vi "pumpsec_new.vi"() -> ()   [LabVIEW 2015]
uses:
  BERTTA.dll
panel:
  out "mA":dbl format="%#_2g"
  out "params":dbl[](array[numeric])
  in  "Time":dbl[](array[numeric])=[4.0, 2.0, 0.0, 0.0, 0.0, 0.0, 0.0, 0.0, 0.0, 0.0]
  in  "Target":dbl[](array[numeric])=[10.0, 2.0, 0.0, 0.0, 0.0, 0.0, 0.0, 0.0, 0.0, 0.0]
  out "Scale":dbl
  in  "Port":i32=10
  in  "reset":i32
  in  "pause":i32
  in  "master":i32
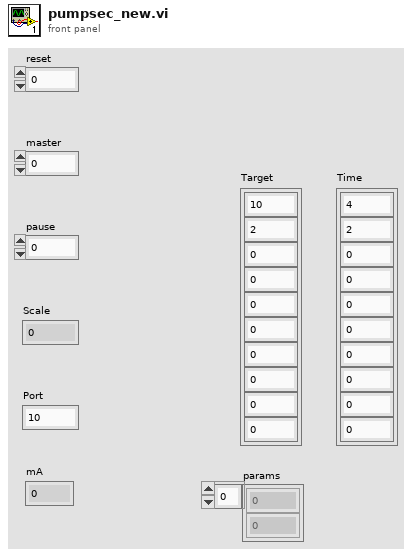
[diagram p1: front panel]
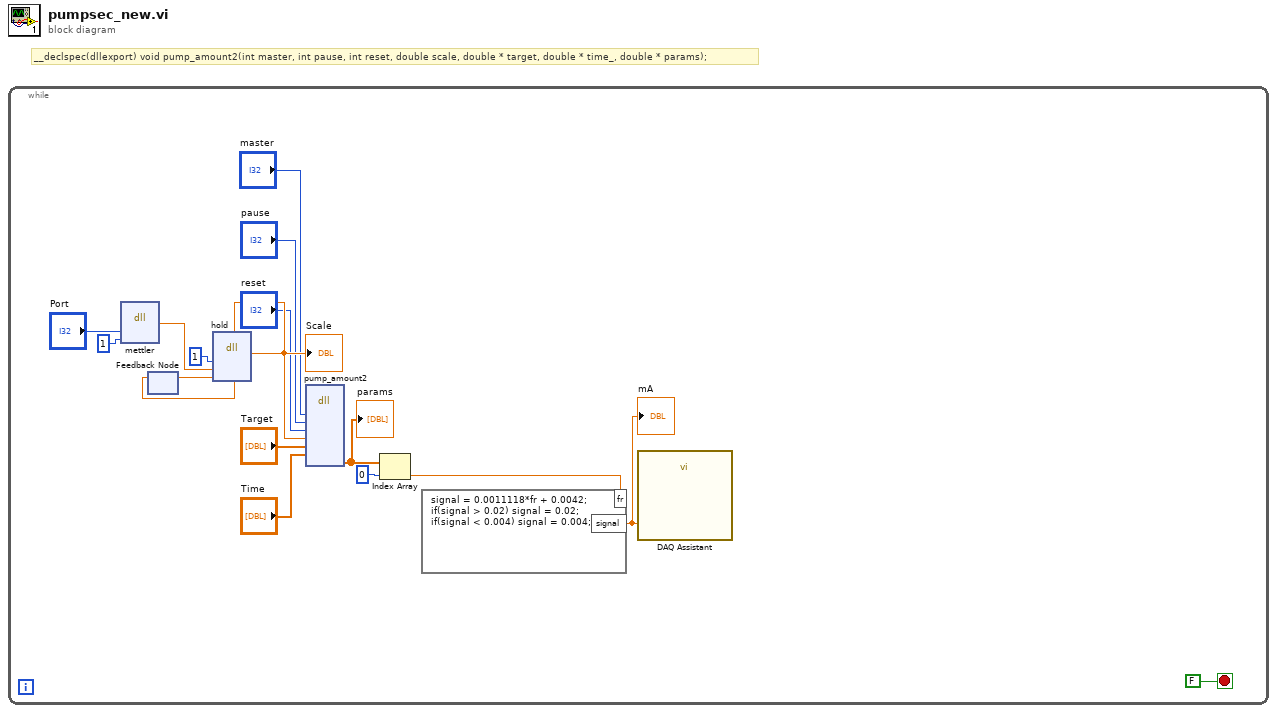
[diagram p0: block diagram]
diagram:
  # "__declspec(dllexport) void pump_amount2(int master, int pause, int reset, double scale, double * target, double * time_, double * params);"
  n1 = while {
    stop <- FALSE stop-if-true
    n2 = dll-call lib="C:/Users/shresplab/OneDrive - Kemira Oyj/Documents/Visual Studio 2017/Projects/Bertta/BERTTA/x64/Debug/BERTTA.dll" fn="mettler"("port"="Port", "msg"=1) -> ("return type"=w10:dbl)  [unwired: 5 in, 2 out]
    n3 = feedback #1() -> (w11:dbl)  [unwired: 1 in]
    n4 = dll-call lib="C:/Users/shresplab/OneDrive - Kemira Oyj/Documents/Visual Studio 2017/Projects/Bertta/BERTTA/x64/Debug/BERTTA.dll" fn="hold"("enable"=1, "in1"=w10, "in2"=w11) -> ("return type"=w15:dbl)  [unwired: 6 in, 2 out]
    "Scale" <- w15
    n5 = feedback-in #1(w15) -> ()
    n6 = dll-call lib="C:/Users/shresplab/OneDrive - Kemira Oyj/Documents/Visual Studio 2017/Projects/Bertta/BERTTA/x64/Debug/BERTTA.dll" fn="pump_amount2"("master"="master", "pause"="pause", "reset"="reset", "scale"=w15, "target"="Target", "time_"="Time") -> ("params"=w6:dbl[])  [unwired: 11 in, 2 out]
    "params" <- w6
    n7 = Index Array(array=w6, index=0) -> (element=w8:dbl)
    n8 = formula code="signal = 0.0011118*fr + 0.0042;\nif(signal > 0.02) signal = 0.02;\nif(signal < 0.004) signal = 0.004;"("fr"=w8) -> ("signal"=w9:dbl)
    "mA" <- w9
    n9 = call "DAQ Assistant"("data"=w9) -> ()  [unwired: 17 in, 2 out]
  }
